vi "TestiLabview.vi"() -> ()   [LabVIEW 2018]
panel:
  out "Image":T1(plugin-control)
  out "Array":cluster{"X Centroid":sgl, "Y Centroid":sgl}[](array[cluster])
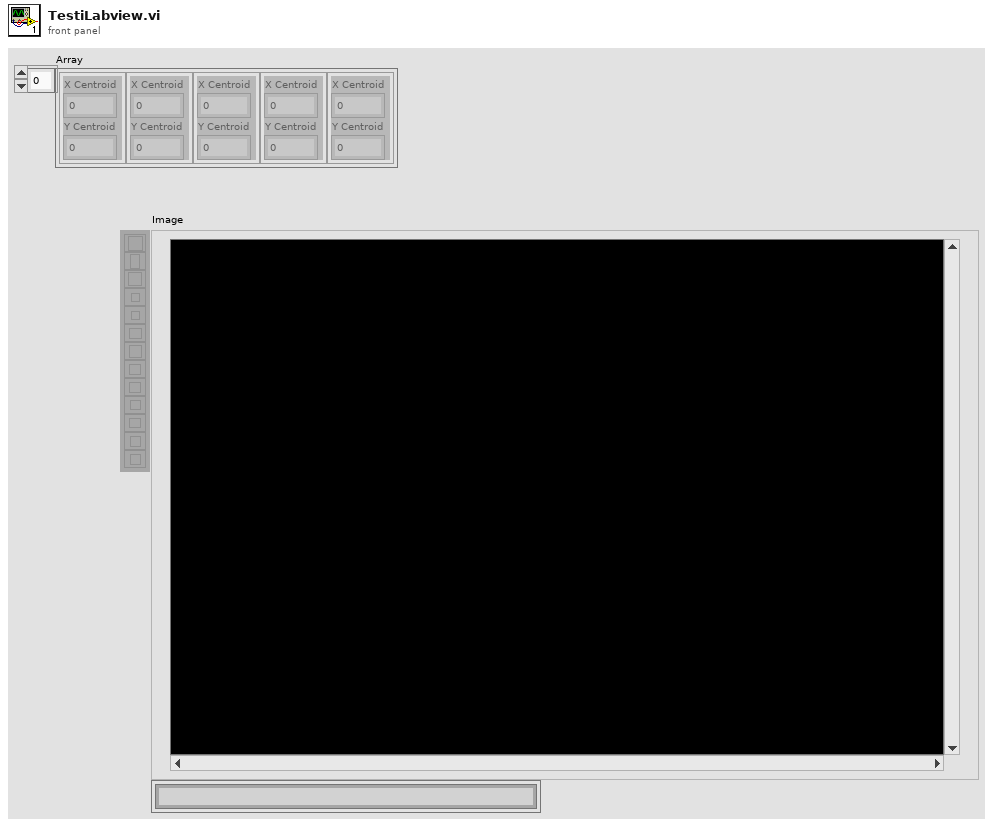
[diagram p1: front panel]
types:
  T1 = typedef "IMAQ Image.ctl" = refnum<image>
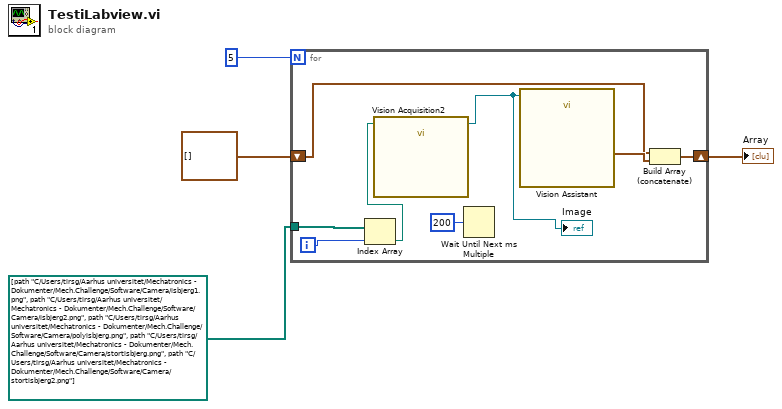
[diagram p0: block diagram]
diagram:
  n1 = for {
    N: 5 -> [_]
    shift-right: [w12] -> w4
    shift-left: cluster{"X Centroid":sgl, "Y Centroid":sgl}[] [] -> [w10]
    tunnel: path[] [path "C:/Users/tirsg/Aarhus universitet/Mechatronics - Dokumenter/Mech.Challenge/Software/Camera/isbjerg1.png", path "C:/Users/tirsg/Aarhus universitet/Mechatronics - Dokumenter/Mech.Challenge/Software/Camera/isbjerg2.png", path "C:/Users/tirsg/Aarhus universitet/Mechatronics - Dokumenter/Mech.Challenge/Software/Camera/polyisbjerg.png", path "C:/Users/tirsg/Aarhus universitet/Mechatronics - Dokumenter/Mech.Challenge/Software/Camera/stortisbjerg.png", path "C:/Users/tirsg/Aarhus universitet/Mechatronics - Dokumenter/Mech.Challenge/Software/Camera/stortisbjerg2.png"] ("appended array") -> [w8]
    i -> [w9]
    n2 = Index Array(array=w8, index=w9) -> (element=w6:path)
    n3 = call "Vision Acquisition2"("Image Path"=w6) -> ("Image Out"=w7:T1)  [unwired: 25 in, 1 out]
    "Image" <- w7
    n4 = Wait Until Next ms Multiple(millisecond multiple=u32 200) -> ()  [unwired: 1 out]
    n5 = call "Vision Assistant"("Image In"=w7) -> ("Centroid (Centroid 1)"=w11:cluster{"X Centroid":sgl, "Y Centroid":sgl})  [unwired: 23 in, 3 out]
    n6 = Build Array (concatenate)(w10, w11) -> (w12:cluster{"X Centroid":sgl, "Y Centroid":sgl}[])
  }
  "Array" <- w4
